vi "Meter Randomize Measurements.vi"(10 "DeviceID":T2) -> (3 "Meter_Measurement Array out":T1[](array[typedef]))   [LabVIEW 2018, in "IED Test Framework.lvlib" / "IED Test.lvclass"]
uses:
  IED Test.lvclass
  <vilib>/ORNL/CSEISMIC DDS/CSEISMIC DDS Base/Data Types/Controls/DeviceID.ctl
  <vilib>/ORNL/CSEISMIC DDS/CSEISMIC DDS Base/Data Types/Meter_Measurement.ctl
  <vilib>/ORNL/CSEISMIC DDS/CSEISMIC DDS Base/CSEISMIC DDS.lvclass
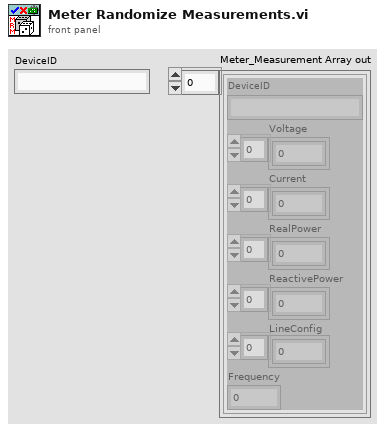
[diagram p1: front panel]
types:
  T1 = typedef "CSEISMIC DDS.lvlib/CSEISMIC DDS.lvclass/Meter_Measurement.ctl" = cluster{"DeviceID":T2, "Voltage":dbl[], "Current":dbl[], "RealPower":dbl[], "ReactivePower":dbl[], "LineConfig":u8[], "Frequency":dbl}
  T2 = typedef "CSEISMIC DDS.lvlib/CSEISMIC DDS.lvclass/DeviceID.ctl" = string
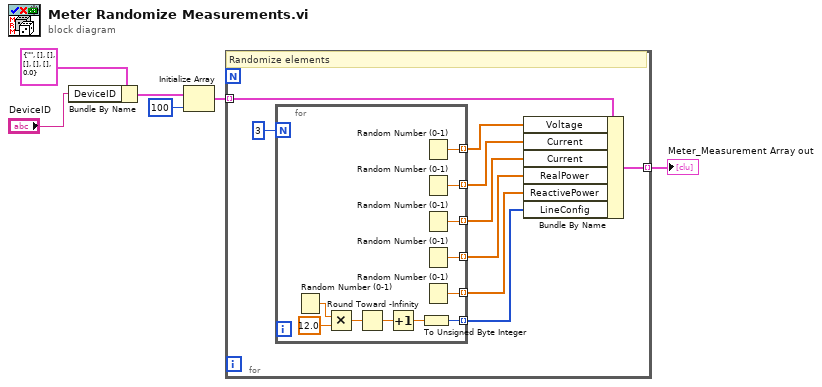
[diagram p0: block diagram]
diagram:
  n1 = Bundle By Name(cluster=T1 {"DeviceID"="", "Voltage"=[], "Current"=[], "RealPower"=[], "ReactivePower"=[], "LineConfig"=[], "Frequency"=0.0} ("Meter_Measurement Array out"), "DeviceID"="DeviceID") -> (w6:T1)
  n2 = Initialize Array(w6, 100 ("dimension size")) -> (w3:T1[])
  n3 = for {
    tunnel: w3 -> [w15] mode=indexing
    tunnel: [w14] -> w1 mode=indexing
    # "Randomize elements"
    n4 = for {
      N: 3 -> [_]
      tunnel: [w26] -> w12 mode=indexing
      tunnel: [w25] -> w11 mode=indexing
      tunnel: [w24] -> w10 mode=indexing
      tunnel: [w23] -> w9 mode=indexing
      tunnel: [w22] -> w8 mode=indexing
      tunnel: [w17] -> w7 mode=indexing
      n5 = Random Number (0-1)() -> (number: 0 to 1=w21:dbl)
      n6 = Multiply(x=w21, y=12.0) -> (x*y=w19:dbl)
      n7 = Round Toward -Infinity(1:w19) -> (0:w18:dbl)
      n8 = Increment(x=w18) -> (x+1=w16:dbl)
      n9 = To Unsigned Byte Integer(number=w16) -> (unsigned 8bit integer=w17:u8)
      n10 = Random Number (0-1)() -> (number: 0 to 1=w26:dbl)
      n11 = Random Number (0-1)() -> (number: 0 to 1=w25:dbl)
      n12 = Random Number (0-1)() -> (number: 0 to 1=w24:dbl)
      n13 = Random Number (0-1)() -> (number: 0 to 1=w23:dbl)
      n14 = Random Number (0-1)() -> (number: 0 to 1=w22:dbl)
    }
    n15 = Bundle By Name(cluster=w15, "Voltage"=w12, "Current"=w11, "Current"=w10, "RealPower"=w9, "ReactivePower"=w8, "LineConfig"=w7) -> (w14:T1)
  }
  "Meter_Measurement Array out" <- w1
